vi "Global 1.vi"() -> ()   [LabVIEW 2014]
panel:
  in  "operand":dbl
  in  "a":dbl
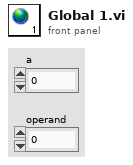
[diagram p1: front panel]
diagram:
